vi "screen for manual mode entry.vi"() -> ()   [LabVIEW 2022 SP3]
panel:
  in  "?":bool
  in  "stop":bool
  in  "?":string
  in  "?":bool=TRUE
  in  "?":bool=TRUE
  in  "Close Button":bool
  # "START NEW\nOPERATION"
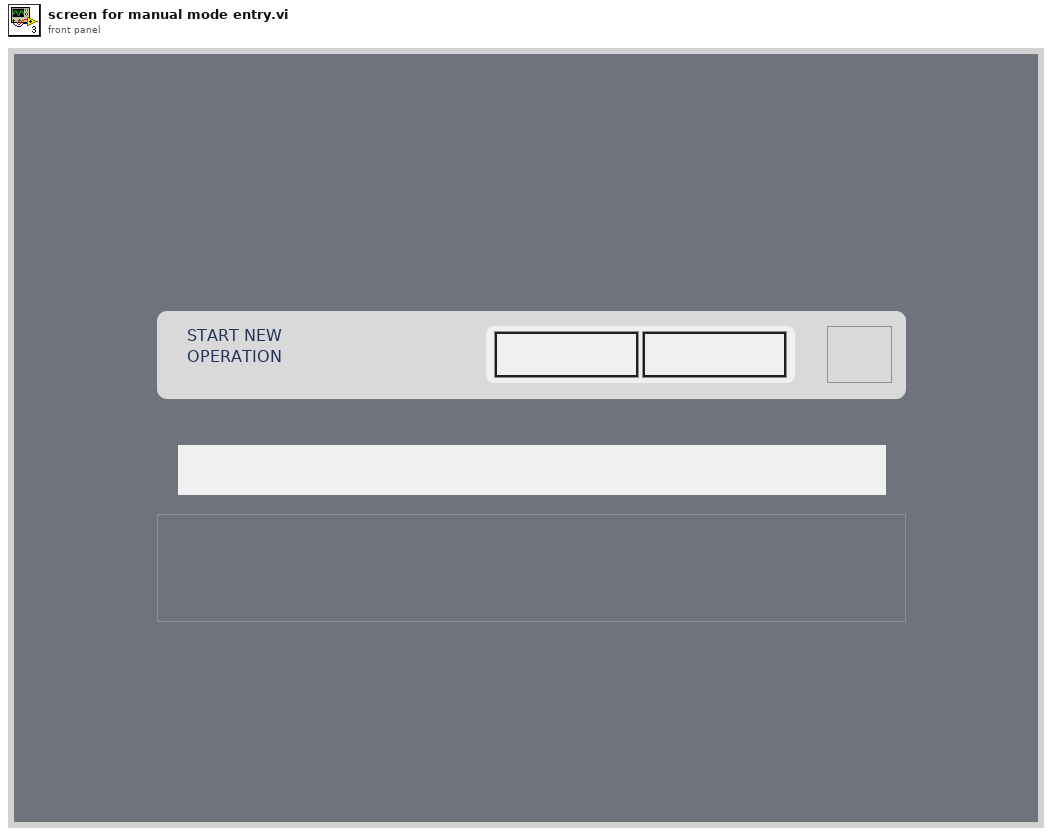
[diagram p1: front panel]
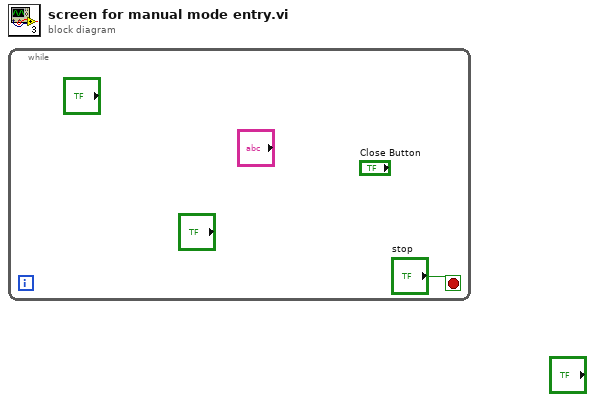
[diagram p0: block diagram]
diagram:
  n1 = while {
    stop <- "stop" stop-if-true
  }
